vi "Demodlator.vi"(8 "error in (no error)":errorcluster, 10 "Waveform in":waveform(dbl), 11 "ISO 14443 B DOWN in":refnum<class "ISO 14443 B DOWN.lvclass">) -> (0 "error out":errorcluster, 2 "Waveform out":waveform(dbl), 3 "ISO 14443 B DOWN out":refnum<class "ISO 14443 B DOWN.lvclass">)   [LabVIEW 2019, in "ISO 14443 B DOWN.lvclass"]
uses:
  ISO 14443 B DOWN.lvclass
  TypeDef/Store.ctl
  ISO 14443 B DOWN.lvclass/ISO 14443 B DOWN.ctl
  <vilib>/addons/Modulation/Analog/support/mod_Set Error Source.vi
  <vilib>/addons/Modulation/Analog/MT Downconvert Passband (Real).vi
  <vilib>/addons/Modulation/Analog/MT Demodulate AM (DSB).vi
  <vilib>/addons/Modulation/Digital/Support/Common/Validators/mod_Generate Filter Coefficients Validate.vi
  <vilib>/addons/Modulation/Digital/General/subVIs/mod_Generate Filter Coefficients.vi
  <vilib>/addons/Modulation/Digital/General/MT Generate ASK system parameters (M).vi
  <vilib>/addons/Modulation/niAMT.lvlib
  <vilib>/addons/Modulation/niDMT.lvlib
  RFID system.lvclass
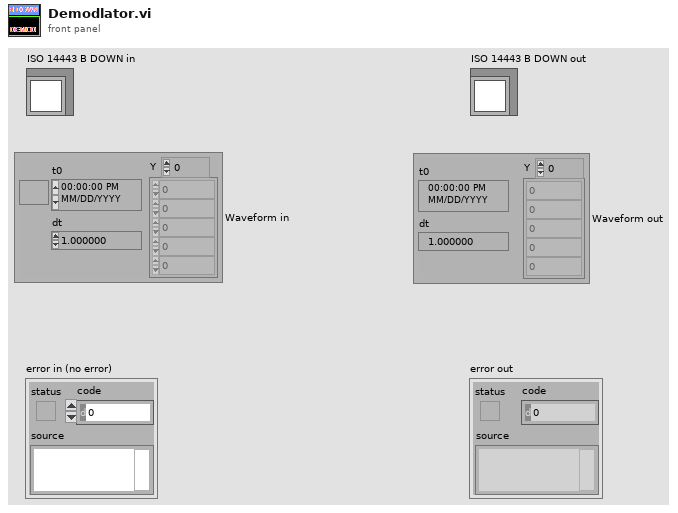
[diagram p1: front panel]
types:
  T1 = typedef "Store.ctl" = enum16{"envelope", "noise", "demSubCar", "CH_frame", "Decode", "demodulate", "in", "out", "sum", "subCarrier", "frame", "command", "encode", "modulate", "encode_UP", "modulate_up", "demod_up", "envelop_up", "sum_up", "out_up", "in_up"}
  T2 = enum16{"none", "Raised Cosine", "Root Raised Cos", "Gaussian"}
  T3 = enum16{"FSK", "PSK", "QAM", "MSK", "PAM", "ASK", "CPM"}
  T4 = cluster{"passband ripple (dB)":dbl, "stopband start (Hz)":dbl, "stopband gain (dB)":dbl, "compute filter stopband ? (T)":bool}
  T5 = typedef "niAMT.lvlib/Complex Data Waveform.ctl" = cluster{"t0":dbl, "dt":dbl, "Y":cdb[]}
  T6 = cluster{"samples per symbol (16)":i32, "symbol map":cdb[]}
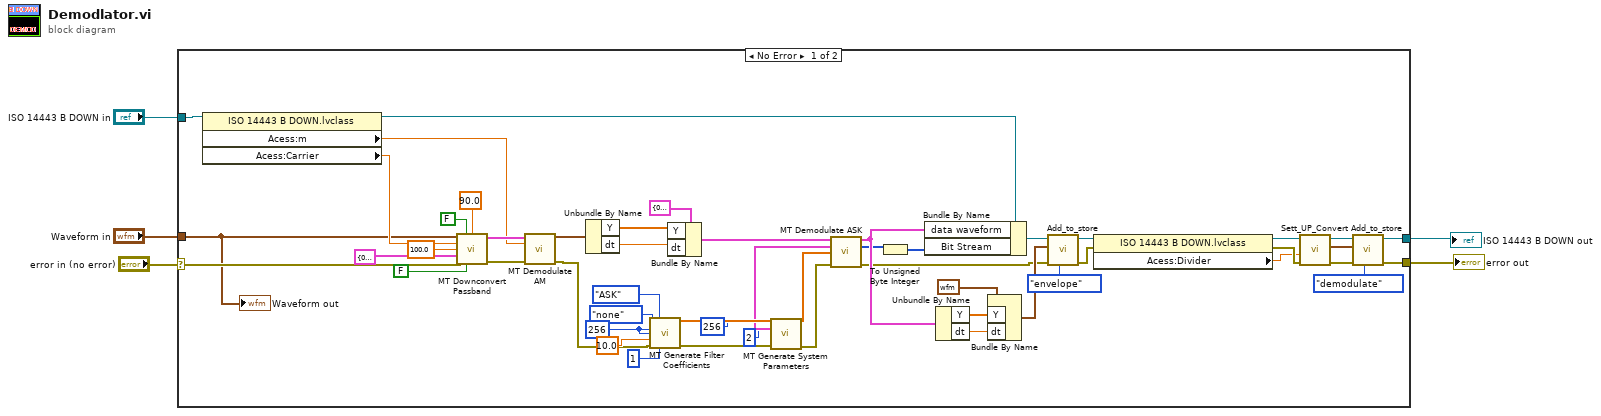
[diagram p0: block diagram]
diagram:
  n1 = case shown="No Error" "error in (no error)" {
    selector: "error in (no error)" -> [w11 w57]
    tunnel: "ISO 14443 B DOWN in" -> [w12 w58]
    tunnel: [w10 w58] -> w4
    tunnel: "Waveform in" -> [w6 _]
    tunnel: [w9 w57] -> w1
    frame No Error {
      w40 = 256 ("pulse shaping samples per symbol (16)")
      n2 = property class="ISO 14443 B DOWN.lvclass"(reference=w12) -> (reference out=w32:refnum<class "ISO 14443 B DOWN.lvclass">, "Acess:m"=w14:dbl, "Acess:Carrier"=w13:dbl)  [unwired: 1 in, 1 out]
      n3 = call-poly <vilib>:"MT Downconvert Passband.vi"("Waveform"=w6, "reset? (F)"=FALSE, "initial phase (deg)"=90.0, "carrier frequency (Hz)"=w13, "passband bandwidth (Hz)"=100.0, "advanced filter parameters"=T4 {"passband ripple (dB)"=0.01, "stopband start (Hz)"=0.0, "stopband gain (dB)"=-96.0, "compute filter stopband ? (T)"=TRUE}, "error in (no error)"=w11, "enable filter (T)"=FALSE) -> ("downconverted waveform (complex baseband)"=w56:T5, "error out"=w55:errorcluster)  [unwired: 4 in, 2 out]
      n4 = call-poly <vilib>:"MT Demodulate AM.vi"("AM modulated waveform"=w56, "modulation index"=w14, "error in (no error)"=w55) -> ("AM demodulated waveform"=w35:waveform(dbl), "error out"=w34:errorcluster)  [unwired: 10 in, 1 out]
      n5 = Unbundle By Name(w35) -> ("Y"=w47:dbl[], "dt"=w48:dbl)
      n6 = call <vilib>:"MT Generate Filter Coefficients.vi"("pulse shaping filter (none)"=T2."none", "modulation type"=T3."ASK", "pulse shaping samples per symbol (16)"=w40, "matched samples per symbol (16)"=w40, "filter parameter"=10.0, "error in (no error)"=w34, "filter length (symbols)"=1) -> ("pulse shaping filter coefficients"=w46:dbl[], "error out"=w44:errorcluster)  [unwired: 7 out]
      n7 = Bundle By Name(cluster=cluster{"t0":dbl, "dt":dbl, "Y":dbl[]} {"t0"=0.0, "dt"=0.0, "Y"=[]} ("AM modulated waveform"), "Y"=w47, "dt"=w48) -> (w49:cluster{"t0":dbl, "dt":dbl, "Y":dbl[]})
      n8 = call-poly <vilib>:"MT Generate System Parameters.vi"("samples per symbol (16)"=256, "M-ASK (2)"=2, "error in (no error)"=w44) -> ("ASK system parameters"=w45:T6, "error out"=w33:errorcluster)  [unwired: 11 out]
      n9 = call <vilib>:"MT Demodulate ASK.vi"("input complex waveform"=w49, "ASK system parameters"=w45, "matched filter coefficients"=w46, "error in (no error)"=w33) -> ("recovered complex waveform"=w27:T5, "output bit stream"=w8:i8[], "error out"=w25:errorcluster)  [unwired: 7 in, 2 out]
      n10 = To Unsigned Byte Integer(number=w8) -> (unsigned 8bit integer=w7:u8[])
      n11 = Bundle By Name(cluster=w32, "data waveform"=w27, "Bit Stream"=w7) -> (w31:refnum<class "ISO 14443 B DOWN.lvclass">)
      n12 = Unbundle By Name(w27) -> ("Y"=w29:cdb[], "dt"=w28:dbl)
      n13 = Bundle By Name(cluster=waveform(cdb) {"t0"=timestamp(0 s since 1904-01-01), "dt"=1.0, "Y"=[]} ("waveform"), "Y"=w29, "dt"=w28) -> (w26:waveform(cdb))
      n14 = call "Add_to_store.vi"("Store"=Store."envelope", "error in (no error)"=w25, "Waveform"=w26, "RFID system in"=w31) -> ("error out"=w17:errorcluster, "RFID system out"=w23:refnum<class "ISO 14443 B DOWN.lvclass">)  [unwired: 6 in]
      n15 = property class="ISO 14443 B DOWN.lvclass"(reference=w23, error in=w17) -> (reference out=w18:refnum<class "ISO 14443 B DOWN.lvclass">, error out=w16:errorcluster, "Acess:Divider"=w15:dbl)
      n16 = call-dynamic "Sett_UP_Convert.vi"("error in (no error)"=w16, "Divider(1)"=w15, "ISO 14443 B DOWN in"=w18) -> ("error out"=w21:errorcluster, "Waveform"=w20:waveform(dbl), "ISO 14443 B DOWN out"=w22:refnum<class "ISO 14443 B DOWN.lvclass">)  [unwired: 6 in]
      n17 = call "Add_to_store.vi"("Store"=Store."demodulate", "error in (no error)"=w21, "Waveform"=w20, "RFID system in"=w22) -> ("error out"=w9:errorcluster, "RFID system out"=w10:refnum<class "ISO 14443 B DOWN.lvclass">)  [unwired: 6 in]
      "Waveform out" <- w6
    }
    frame Error {
    }
  }
  "error out" <- w1
  "ISO 14443 B DOWN out" <- w4
